vi "Keep BMS in load mode message.vi"(7 "timeout in ms (-1)":i32=-1, 8 "error in":errorcluster, 9 "Error Queue":refnum<queue>, 10 "Shutdown Notifier":refnum<notifier>, 11 "CAN Session In":T1) -> (2 "Exit?":bool, 3 "CAN Session Out":T1)   [LabVIEW 2016]
uses:
  Program Files (x86)/National Instruments/LabVIEW 2016/examples/robotics/EPOS2 CANOpen Driver/Low Level VIs/Typedefs/CAN Refnum.ctl
  Program Files (x86)/National Instruments/LabVIEW 2016/examples/robotics/EPOS2 CANOpen Driver/Low Level VIs/Typedefs/CAN Session Pointer.ctl
  Program Files (x86)/National Instruments/LabVIEW 2016/examples/robotics/EPOS2 CANOpen Driver/Low Level VIs/Typedefs/CAN Communication References.ctl
  Program Files (x86)/National Instruments/LabVIEW 2016/examples/robotics/EPOS2 CANOpen Driver/Low Level VIs/Typedefs/kill process notifier array.ctl
  Program Files (x86)/National Instruments/LabVIEW 2016/examples/robotics/EPOS2 CANOpen Driver/Low Level VIs/Typedefs/Write Queue.ctl
  Program Files (x86)/National Instruments/LabVIEW 2016/examples/robotics/EPOS2 CANOpen Driver/Low Level VIs/Typedefs/FPGA CAN Frame Cluster.ctl
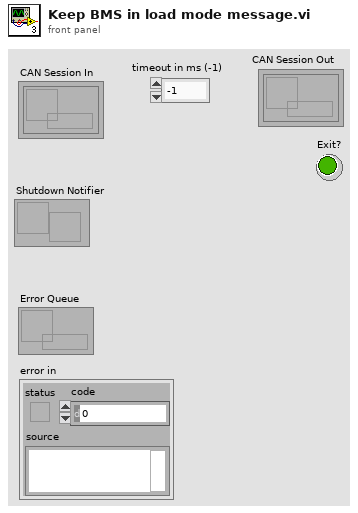
[diagram p1: front panel]
types:
  T1 = typedef "CAN Refnum.ctl" = refnum<k1>
  T2 = typedef "Stage Request Status.ctl" = cluster{"precharge done":bool, "staging ack":bool, "active request":bool}
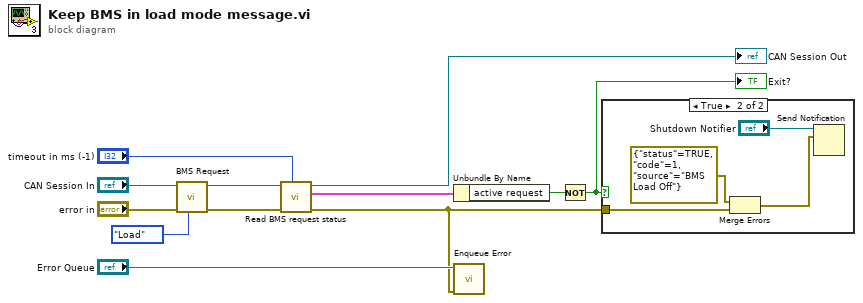
[diagram p0: block diagram]
diagram:
  n1 = call "BMS Request.vi"("Request"=enum16{"Empty", "Load", "Staging"}."Load", "error in"="error in", "CAN Session In"="CAN Session In") -> ("error out"=w11:errorcluster, "CAN Session Out"=w7:T1)  [unwired: 7 in]
  n2 = call "Read BMS request status.vi"("timeout in ms (-1)"="timeout in ms (-1)", "error in"=w11, "CAN Session In"=w7) -> ("error out"=w2:errorcluster, "Stage Request Status"=w9:T2, "CAN Session Out"=→"CAN Session Out":T1)  [unwired: 6 in]
  n3 = Unbundle By Name(w9) -> ("active request"=w8:bool)
  n4 = call "Enqueue Error.vi"("error in"=w2, "Error Queue"="Error Queue") -> ()  [unwired: 10 in]
  n5 = Not(x=w8) -> (.not. x?=w1:bool)
  "Exit?" <- w1
  n6 = case shown="True" w1 {
    tunnel: w2 -> [_ w14]
    frame False {
    }
    frame True {
      n7 = Merge Errors(errorcluster {"status"=TRUE, "code"=1, "source"="BMS Load Off"} ("error constant"), w14) -> (w13:errorcluster)
      n8 = Send Notification(notification=w13, notifier="Shutdown Notifier") -> ()  [unwired: 1 in, 2 out]
    }
  }
